vi "main_new2.vi"() -> ()   [LabVIEW 2019]
uses:
  Controls/data.ctl
  Estats.ctl
panel:
  out "Pict Ring 2":u16(ring)
  in  "Prova":bool
  out "Diners":string
  in  "Stop Button":bool
  out "Diàleg":string
  out "Canvi":string
  in  "Orange":bool
  in  "Lemond":bool
  in  "Apple":bool
  in  "50cents":bool
  in  "20cents":bool
  in  "10cents":bool
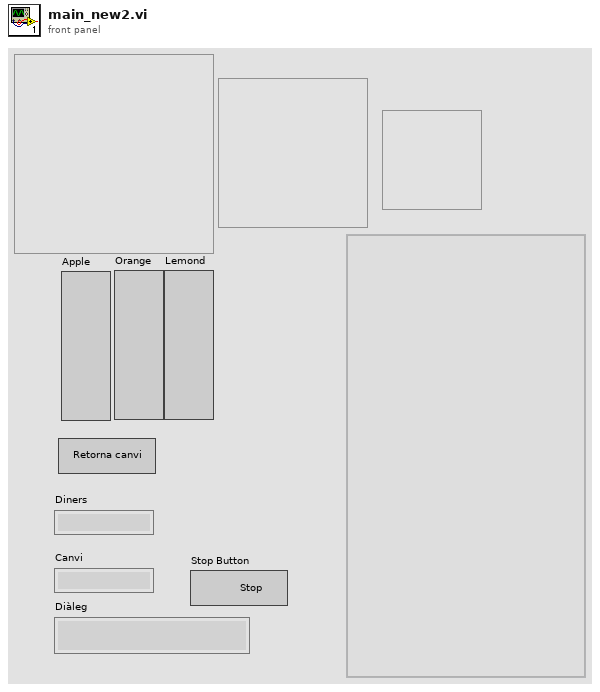
[diagram p1: front panel]
types:
  T1 = typedef "Estats.ctl" = enum16{"Init", "Wait for Event", "Exit", "Return Money", "Lemond", "Apple", "Orange", "Deliver", "50cents", "20cents", "10cents"}
  T2 = typedef "data.ctl" = cluster{"Diners":dbl, "Han triat veguda":bool}
  T3 = enum8{"Enabled", "Disabled", "Disabled and Grayed Out"}
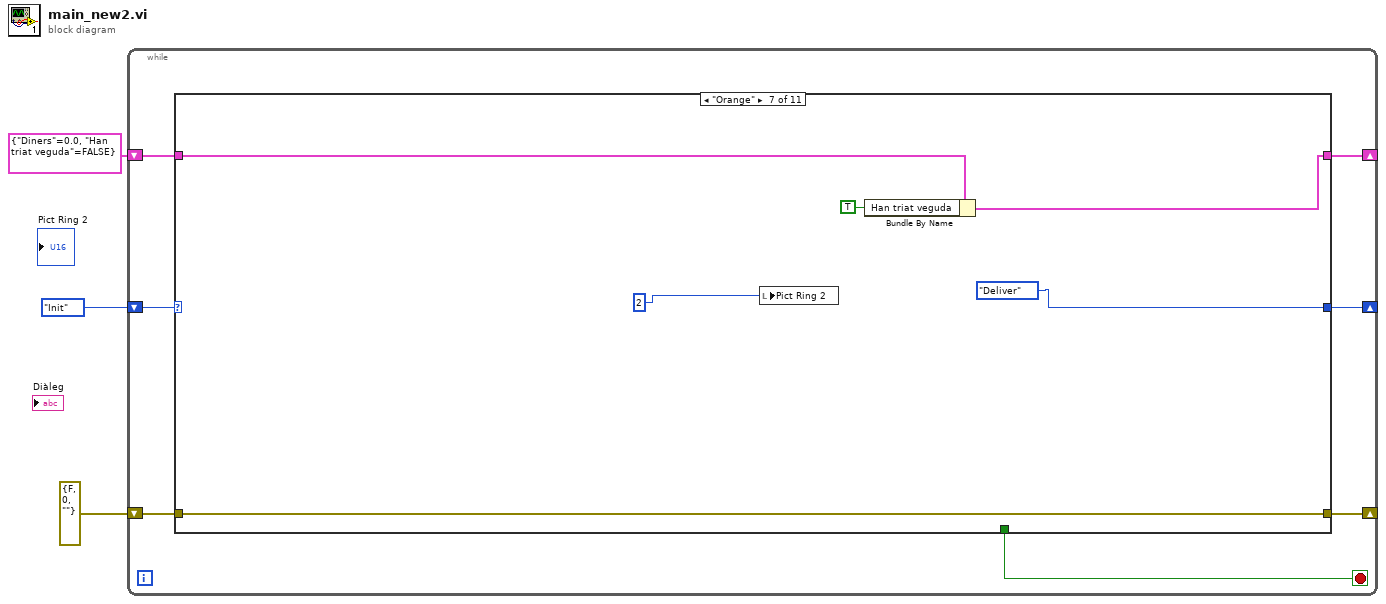
[diagram p0: block diagram]
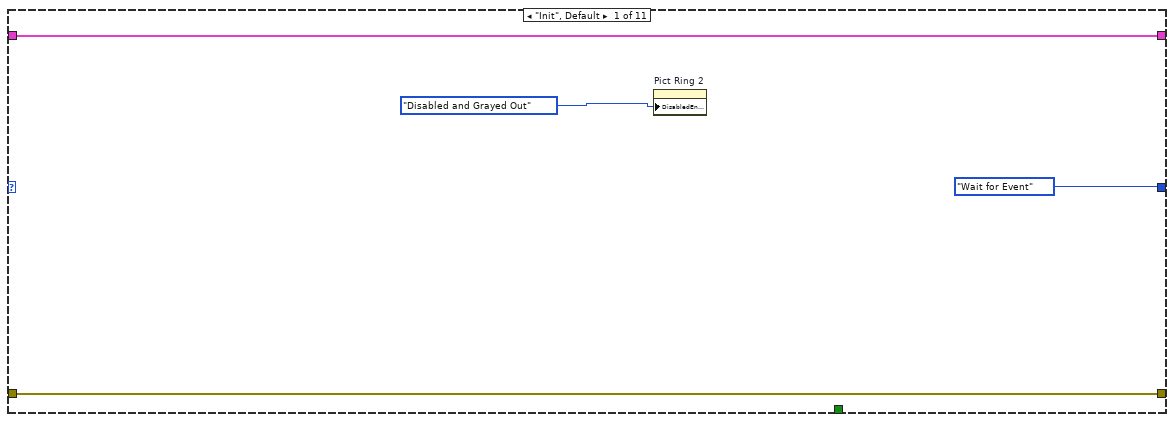
[diagram p2: hidden frame]
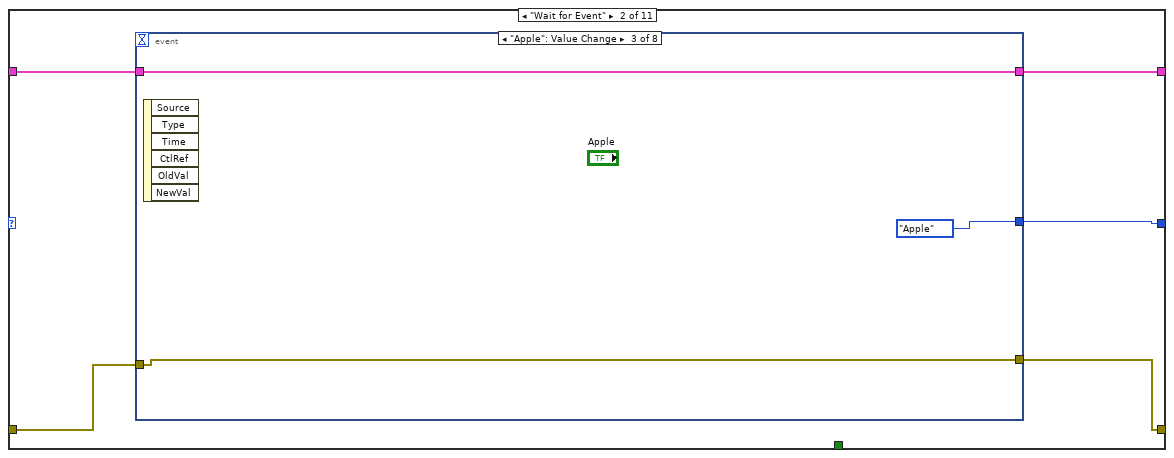
[diagram p3: hidden frame]
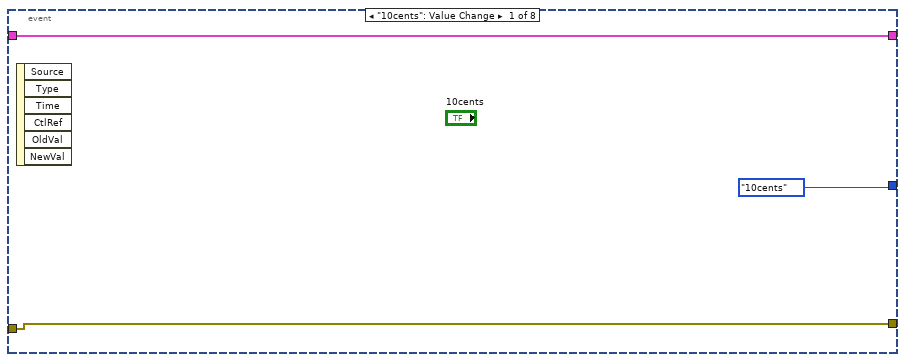
[diagram p4: hidden frame]
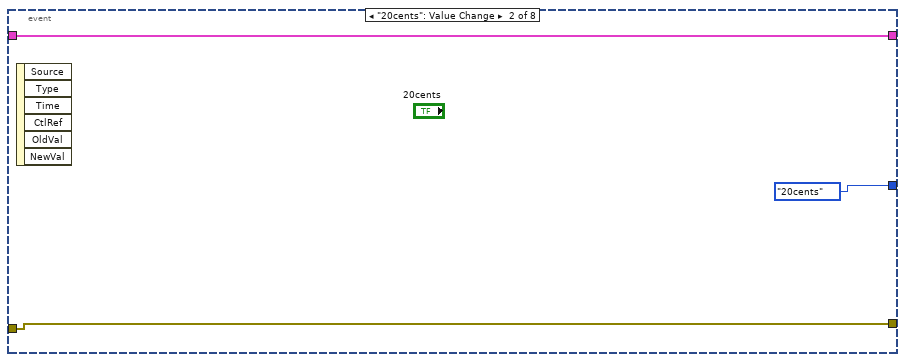
[diagram p5: hidden frame]
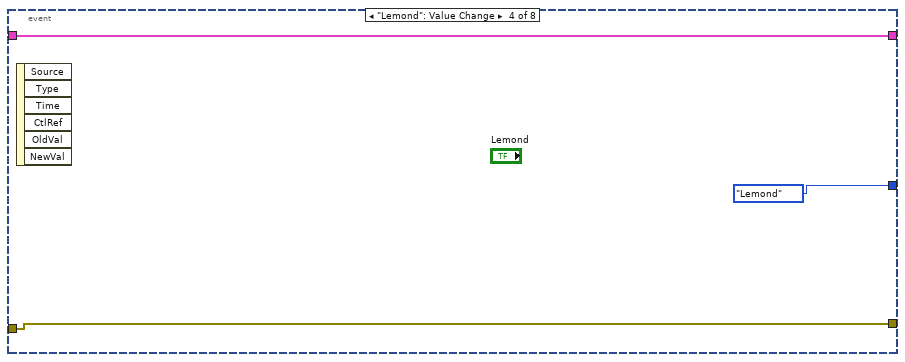
[diagram p6: hidden frame]
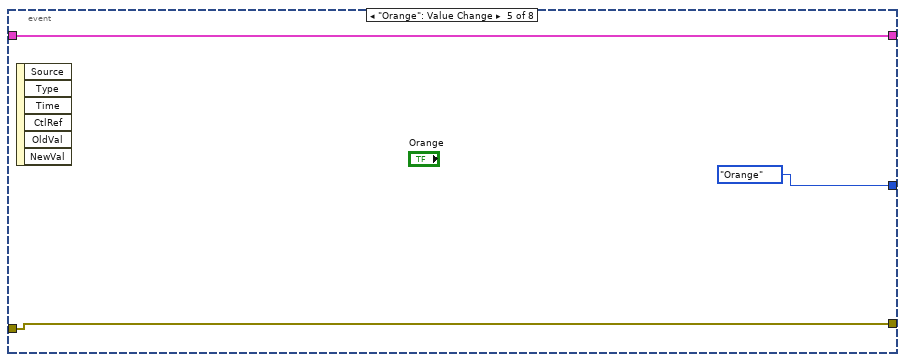
[diagram p7: hidden frame]
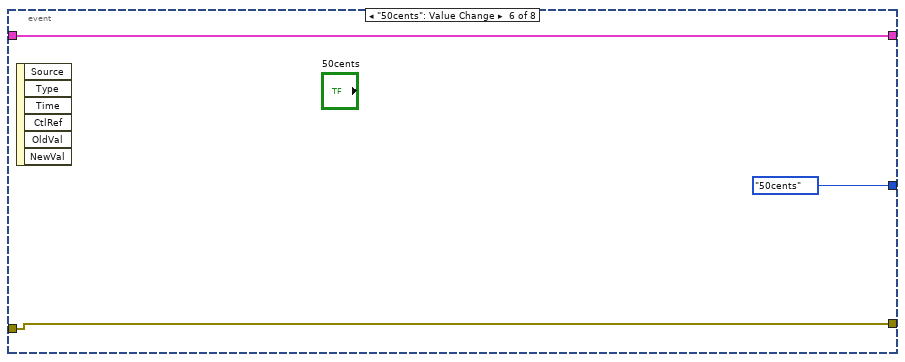
[diagram p8: hidden frame]
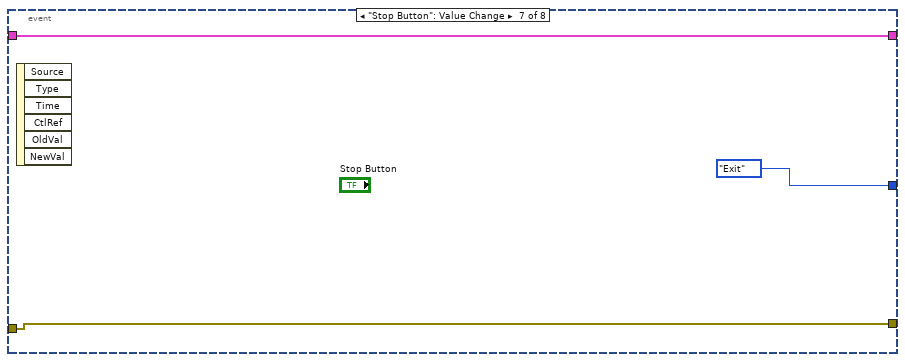
[diagram p9: hidden frame]
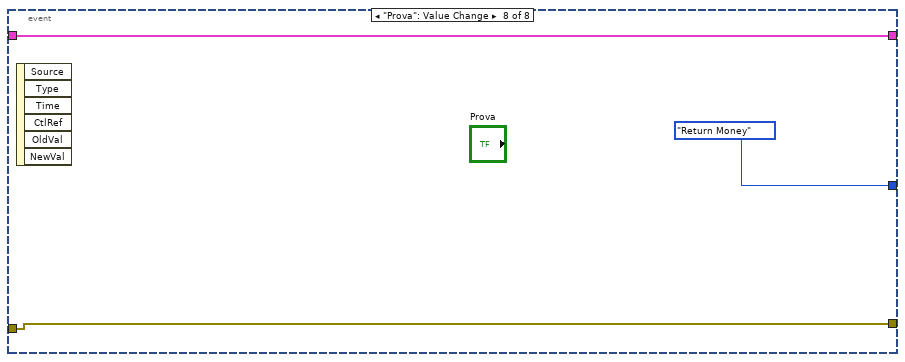
[diagram p10: hidden frame]
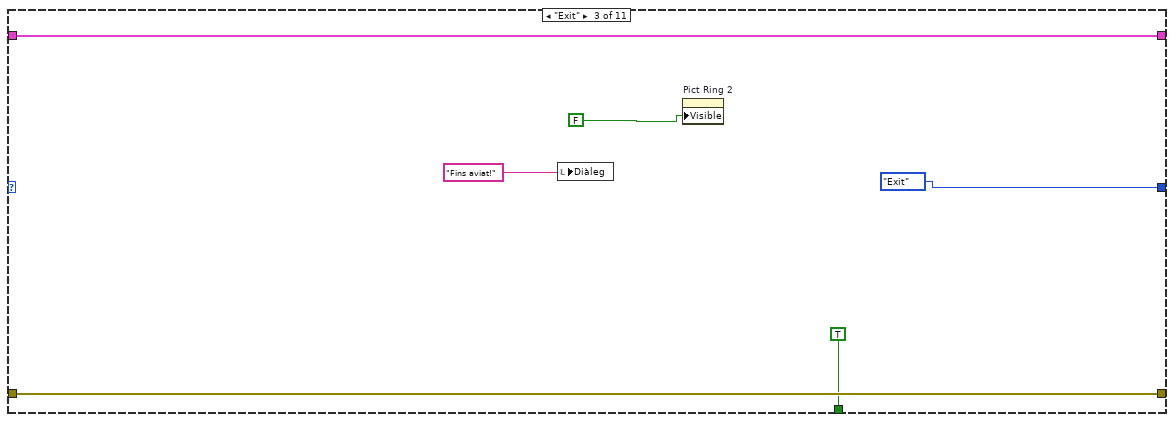
[diagram p11: hidden frame]
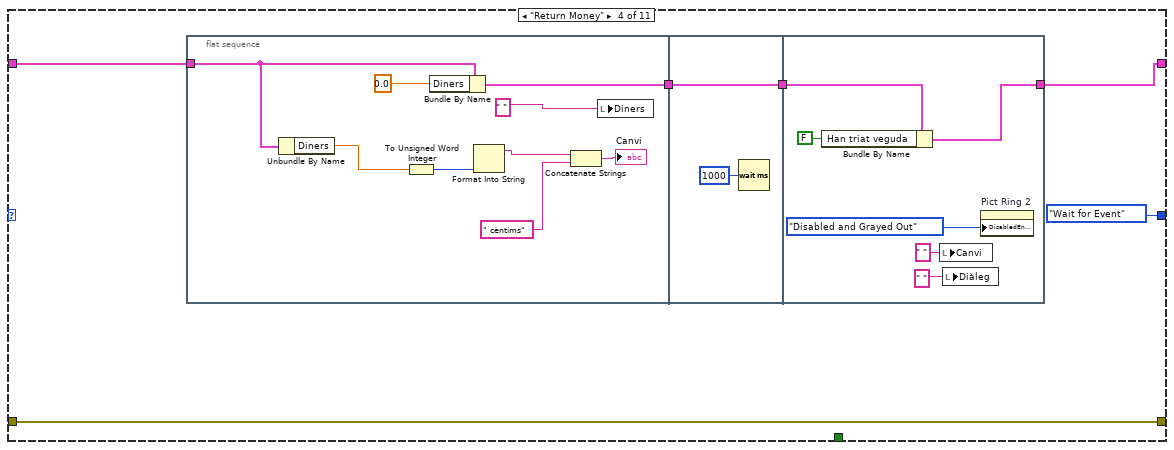
[diagram p12: hidden frame]
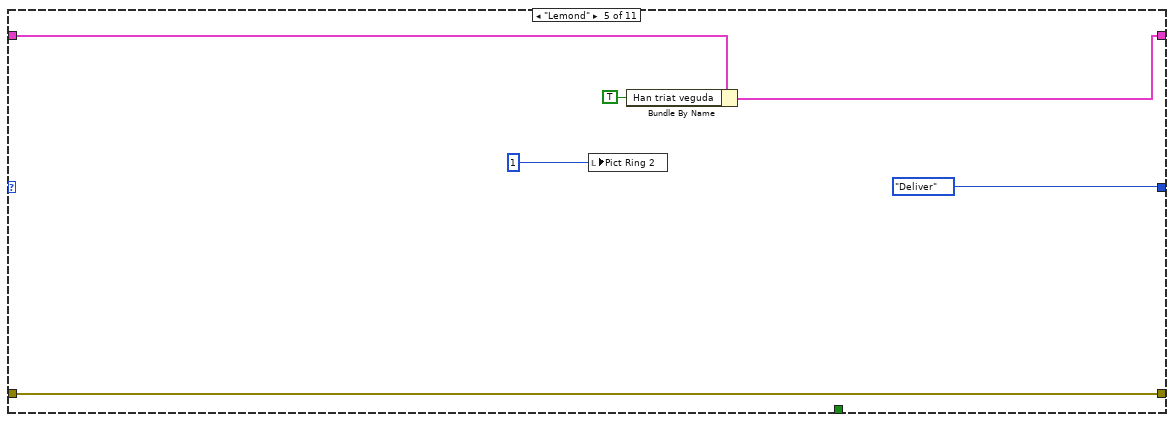
[diagram p13: hidden frame]
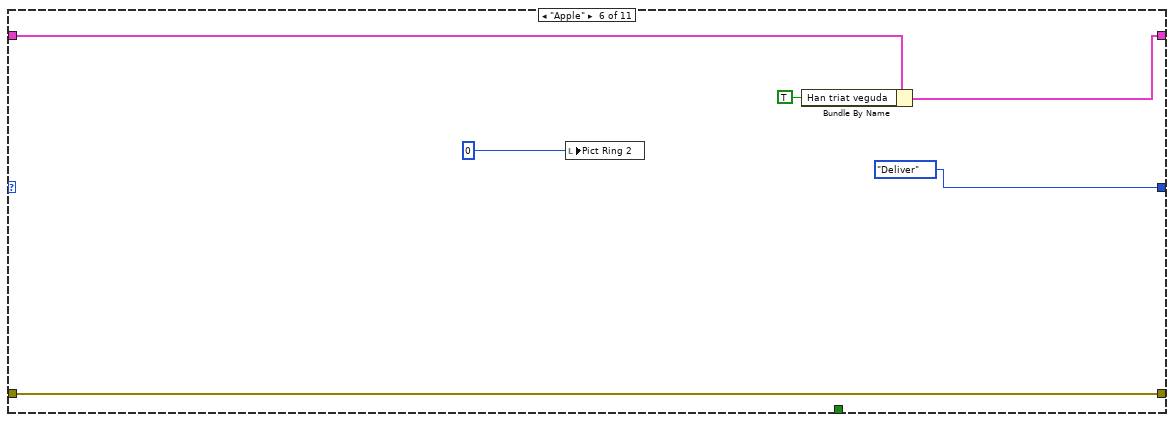
[diagram p14: hidden frame]
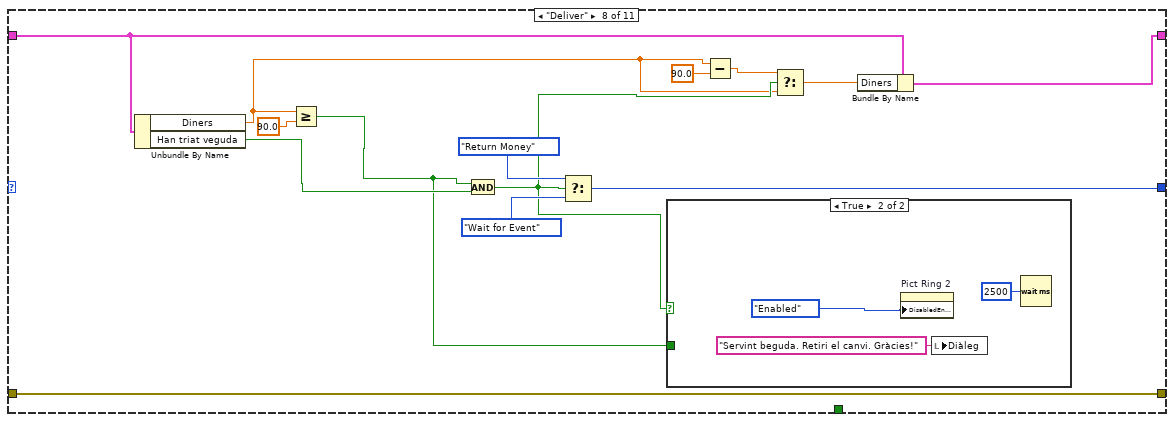
[diagram p15: hidden frame]
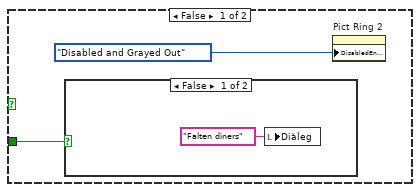
[diagram p16: hidden frame]
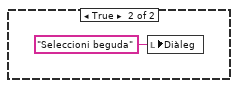
[diagram p17: hidden frame]
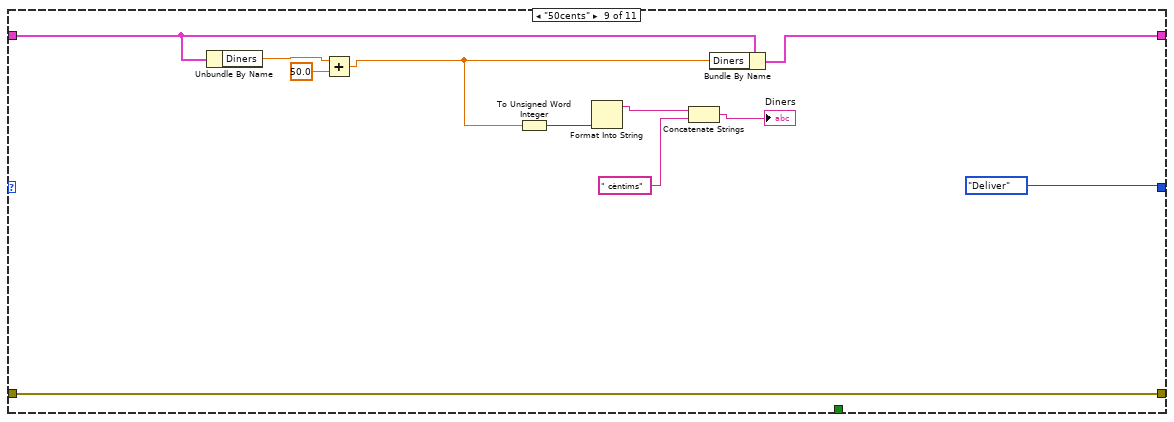
[diagram p18: hidden frame]
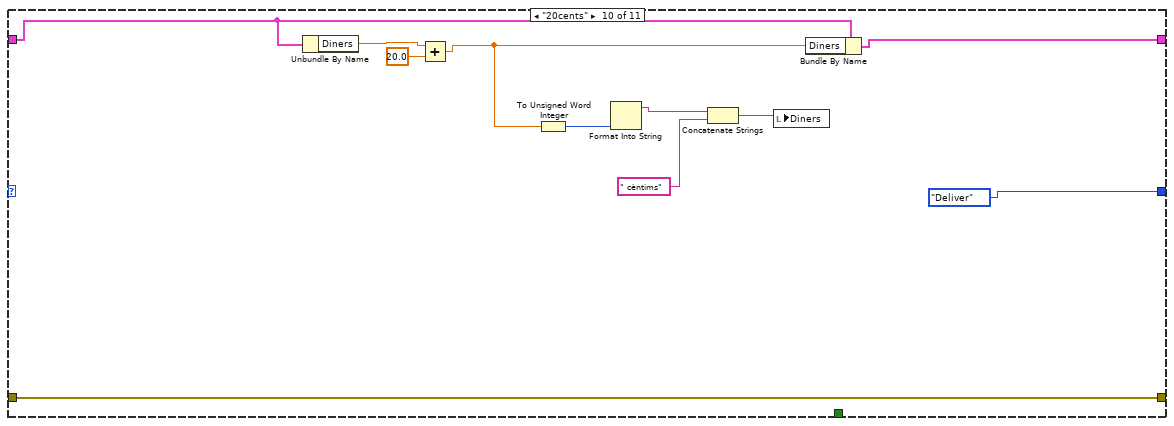
[diagram p19: hidden frame]
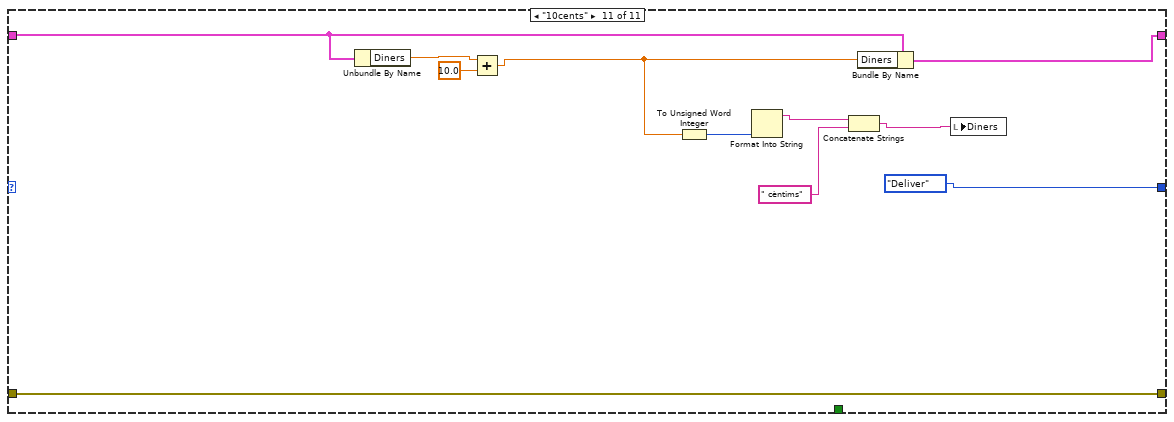
[diagram p20: hidden frame]
diagram:
  n1 = while {
    shift-right: [w5] -> _
    shift-left: Estats."Init" ("Enum") -> [w10]
    shift-right: [w6] -> _
    shift-left: T2 {"Diners"=0.0, "Han triat veguda"=FALSE} ("Cluster") -> [w9]
    shift-right: [w7] -> _
    shift-left: errorcluster {"status"=FALSE, "code"=0, "source"=""} ("error constant") -> [w8]
    stop <- w4 stop-if-true
    n2 = case shown="\"Orange\"" w10 {
      tunnel: w9 -> [w14 w18 w48 w53 w76 w81 w87 w99 w118 w129 w140]
      tunnel: w8 -> [w12 w17 w47 w54 w77 w83 w89 w101 w121 w132 w143]
      tunnel: [w12 w16 w47 w54 w77 w83 w89 w101 w121 w132 w143] -> w7
      tunnel: [w14 w19 w48 w52 w75 w80 w86 w98 w117 w128 w139] -> w6
      tunnel: [Estats."Wait for Event" ("Enum") w15 Estats."Exit" ("Enum") Estats."Wait for Event" ("Enum") Estats."Deliver" ("Enum") Estats."Deliver" ("Enum") Estats."Deliver" ("Enum") w102 Estats."Deliver" ("Enum") Estats."Deliver" ("Enum") Estats."Deliver" ("Enum")] -> w5
      tunnel: [_ _ TRUE ("stop") _ _ _ _ _ _ _ _] -> w4
      frame "Init", Default {
        n3 = property on="Pict Ring 2" class="Ring (strict)"("DisabledEnum"=T3."Disabled and Grayed Out" ("Disabled")) -> ()  [unwired: 2 in, 2 out]
      }
      frame "Wait for Event" {
        n4 = event shown="[2] \"Apple\": Value Change" {
          selector: _ -> [_ _ _ _ _ _ _ _]
          dyn-events: _ -> [_ _ _ _ _ _ _ _]
          timeout: _ -> [_ _ _ _ _ _ _ _]
          tunnel: [w21 w24 w26 w29 w32 w35 w38 w41] -> w19
          tunnel: w18 -> [w21 w24 w26 w29 w32 w35 w38 w41]
          tunnel: w17 -> [w20 w23 w27 w30 w33 w36 w39 w42]
          tunnel: [w20 w23 w27 w30 w33 w36 w39 w42] -> w16
          tunnel: [Estats."10cents" ("Enum") Estats."20cents" ("Enum") Estats."Apple" ("Enum") Estats."Lemond" ("Enum") Estats."Orange" ("Enum") Estats."50cents" ("Enum") Estats."Exit" ("Enum") Estats."Return Money" ("Enum")] -> w15
          event "10cents": Value Change {
            n5 = event-data() -> ()  [unwired: 1 in, 6 out]
          }
          event "20cents": Value Change {
            n6 = event-data() -> ()  [unwired: 1 in, 6 out]
          }
          event "Apple": Value Change {
            n7 = event-data() -> ()  [unwired: 1 in, 6 out]
          }
          event "Lemond": Value Change {
            n8 = event-data() -> ()  [unwired: 1 in, 6 out]
          }
          event "Orange": Value Change {
            n9 = event-data() -> ()  [unwired: 1 in, 6 out]
          }
          event "50cents": Value Change {
            n10 = event-data() -> ()  [unwired: 1 in, 6 out]
          }
          event "Stop Button": Value Change {
            n11 = event-data() -> ()  [unwired: 1 in, 6 out]
          }
          event "Prova": Value Change {
            n12 = event-data() -> ()  [unwired: 1 in, 6 out]
          }
        }
      }
      frame "Exit" {
        n13 = local write "Diàleg"("Fins aviat!" ("Estat")) -> ()
        n14 = property on="Pict Ring 2" class="Ring (strict)"("Visible"=FALSE) -> ()  [unwired: 2 in, 2 out]
      }
      frame "Return Money" {
        n15 = flat-sequence {
          tunnel: w53 -> [w62]
          tunnel: [w61] -> w51
          tunnel: w51 -> [w66]
          tunnel: [w66] -> w50
          tunnel: [w70] -> w52
          tunnel: w50 -> [w68]
          frame #0 {
            n16 = Unbundle By Name(w62) -> ("Diners"=w59:dbl)
            n17 = To Unsigned Word Integer(number=w59) -> (unsigned 16bit integer=w60:u16)
            n18 = Bundle By Name(cluster=w62, "Diners"=0.0) -> (w61:T2)
            n19 = Format Into String(w60) -> (resulting string=w63:string)  [unwired: 3 in, 1 out]
            n20 = Concatenate Strings(w63, " cèntims" ("string")) -> (→"Canvi":string)
            n21 = local write "Diners"(" " ("Canvi")) -> ()
          }
          frame #1 {
            n22 = Wait (ms)(milliseconds to wait=u32 1000) -> ()  [unwired: 1 out]
          }
          frame #2 {
            n23 = Bundle By Name(cluster=w68, "Han triat veguda"=FALSE) -> (w70:T2)
            n24 = local write "Canvi"(" " ("Canvi")) -> ()
            n25 = local write "Diàleg"(" " ("Canvi")) -> ()
            n26 = property on="Pict Ring 2" class="Ring (strict)"("DisabledEnum"=T3."Disabled and Grayed Out" ("Disabled")) -> ()  [unwired: 2 in, 2 out]
          }
        }
      }
      frame "Lemond" {
        n27 = local write "Pict Ring 2"(u16 1 ("Ring")) -> ()
        n28 = Bundle By Name(cluster=w76, "Han triat veguda"=TRUE) -> (w75:T2)
      }
      frame "Apple" {
        n29 = local write "Pict Ring 2"(u16 0 ("Ring")) -> ()
        n30 = Bundle By Name(cluster=w81, "Han triat veguda"=TRUE) -> (w80:T2)
      }
      frame "Orange" {
        n31 = local write "Pict Ring 2"(u16 2 ("Ring")) -> ()
        n32 = Bundle By Name(cluster=w87, "Han triat veguda"=TRUE) -> (w86:T2)
      }
      frame "Deliver" {
        n33 = Unbundle By Name(w99) -> ("Diners"=w92:dbl, "Han triat veguda"=w100:bool)
        n34 = Greater Or Equal?(x=w92, y=90.0 ("x")) -> (x >= y?=w91:bool)
        n35 = And(x=w91, y=w100) -> (x .and. y?=w94:bool)
        n36 = Select(t=Estats."Return Money" ("Enum"), s=w94, f=Estats."Wait for Event" ("Enum")) -> (s? t:f=w102:T1)
        n37 = case shown="True" w94 {
          tunnel: w91 -> [w106 _]
          frame False {
            n38 = case shown="False" w106 {
              frame False {
                n39 = local write "Diàleg"("Falten diners" ("Diàleg")) -> ()
              }
              frame True {
                n40 = local write "Diàleg"("Seleccioni beguda" ("Diàleg")) -> ()
              }
            }
            n41 = property on="Pict Ring 2" class="Ring (strict)"("DisabledEnum"=T3."Disabled and Grayed Out" ("Disabled")) -> ()  [unwired: 2 in, 2 out]
          }
          frame True {
            n42 = property on="Pict Ring 2" class="Ring (strict)"("DisabledEnum"=T3."Enabled" ("Disabled")) -> ()  [unwired: 2 in, 2 out]
            n43 = local write "Diàleg"("Servint beguda. Retiri el canvi. Gràcies!" ("Estat")) -> ()
            n44 = Wait (ms)(milliseconds to wait=u32 2500) -> ()  [unwired: 1 out]
          }
        }
        n45 = Subtract(x=w92, y=90.0) -> (x-y=w96:dbl)
        n46 = Select(t=w96, s=w94, f=w92) -> (s? t:f=w97:dbl)
        n47 = Bundle By Name(cluster=w99, "Diners"=w97) -> (w98:T2)
      }
      frame "50cents" {
        n48 = Unbundle By Name(w118) -> ("Diners"=w119:dbl)
        n49 = Add(x=w119, y=50.0) -> (x+y=w113:dbl)
        n50 = To Unsigned Word Integer(number=w113) -> (unsigned 16bit integer=w114:u16)
        n51 = Format Into String(w114) -> (resulting string=w112:string)  [unwired: 3 in, 1 out]
        n52 = Concatenate Strings(w112, " cèntims" ("string")) -> (→"Diners":string)
        n53 = Bundle By Name(cluster=w118, "Diners"=w113) -> (w117:T2)
      }
      frame "20cents" {
        n54 = Unbundle By Name(w129) -> ("Diners"=w130:dbl)
        n55 = Add(x=w130, y=20.0) -> (x+y=w124:dbl)
        n56 = To Unsigned Word Integer(number=w124) -> (unsigned 16bit integer=w126:u16)
        n57 = Format Into String(w126) -> (resulting string=w125:string)  [unwired: 3 in, 1 out]
        n58 = Concatenate Strings(w125, " cèntims" ("string")) -> (w123:string)
        n59 = local write "Diners"(w123) -> ()
        n60 = Bundle By Name(cluster=w129, "Diners"=w124) -> (w128:T2)
      }
      frame "10cents" {
        n61 = Unbundle By Name(w140) -> ("Diners"=w141:dbl)
        n62 = Add(x=w141, y=10.0) -> (x+y=w135:dbl)
        n63 = To Unsigned Word Integer(number=w135) -> (unsigned 16bit integer=w137:u16)
        n64 = Format Into String(w137) -> (resulting string=w138:string)  [unwired: 3 in, 1 out]
        n65 = Concatenate Strings(w138, " cèntims" ("string")) -> (w134:string)
        n66 = Bundle By Name(cluster=w140, "Diners"=w135) -> (w139:T2)
        n67 = local write "Diners"(w134) -> ()
      }
    }
  }
